vi "PythonNode_AddTwoDoubles_timed.vi"() -> ()   [LabVIEW 2020]
doc: "This example demonstrates how to call a Python function and pass doubles as arguments. It uses a python function to compute the sum of two doubles."
uses:
  Program Files (x86)/National Instruments/LabVIEW 2020/examples/Connectivity/Python/support/PythonVersionsEnum.ctl
  <vilib>/Utility/High Resolution Relative Seconds.vi
panel:
  out "Time (us)":dbl
  out "Time (ms)":dbl format="%_19f"
  out "error out":errorcluster
  out "a + b":dbl
  in  "b":dbl=1.0
  in  "a":dbl=41.0
  in  "error in (no error)":errorcluster
  in  "Python version":T1
  # "Overview: Demonstrates how to call a Python function and pass doubles as arguments.\nRequirements: Python 2.7 or 3.6 with the same bitness as LabVIEW.\nInstructions:\n1. Set the Python version to the version of Python you want to execute code in.\n2. Run the VI. You should see the result of adding \"a\" and \"b\" in the indicator \"a + b\".\n3. See comments on the block diagram of this VI and in \"ExamplePythonModule.py\" for more information about how the call python node passes arguments and handles return values."
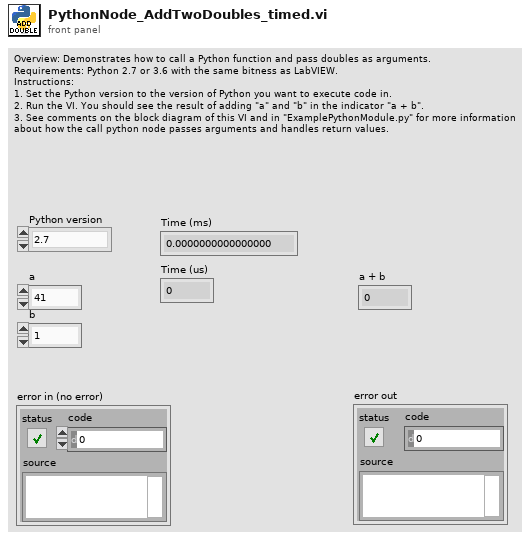
[diagram p1: front panel]
types:
  T1 = typedef "PythonVersionsEnum.ctl" = enum16{"2.7", "3.6"}
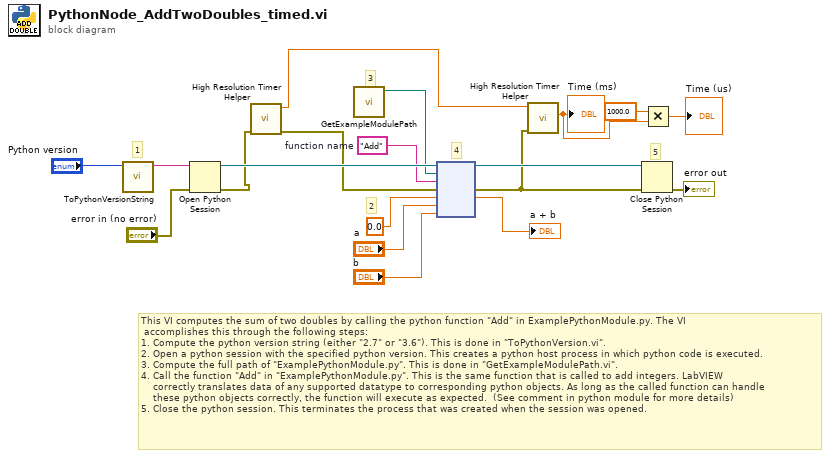
[diagram p0: block diagram]
diagram:
  w14 = "Add"  # function name
  # "5"
  # "4"
  # "2"
  # "3"
  # "1"
  # "This VI computes the sum of two doubles by calling the python function \"Add\" in ExamplePythonModule.py. The VI\n accomplishes this through the following steps:\n1. Compute the python version string (either \"2.7\" or \"3.6\"). This is done in \"ToPythonVersion.vi\". \n2. Open a python session with the specified python version. This creates a python host process in which python code is executed.\n3. Compute the full path of \"ExamplePythonModule.py\". This is done in \"GetExampleModulePath.vi\".\n4. Call the function \"Add\" in \"ExamplePythonModule.py\". This is the same function that is called to add integers. LabVIEW \n    correctly translates data of any supported datatype to corresponding python objects. As long as the called function can handle\n    these python objects correctly, the function will execute as expected.  (See comment in python module for more details)\n5. Close the python session. This terminates the process that was created when the session was opened."
  n1 = call "ToPythonVersionString.vi"("python version"="Python version") -> ("python version string"=w19:string)  [unwired: 10 in]
  n2 = Open Python Session(python version=w19, 3:"error in (no error)") -> (session out=w16:refnum<k35>, error out=w7:errorcluster)  [unwired: 1 in]
  n3 = call "High Resolution Timer Helper.vi"("error in (no error)"=w7) -> ("error out"=w1:errorcluster, "Current Time"=w5:dbl)  [unwired: 8 in, 1 out]
  n4 = call "GetExampleModulePath.vi"() -> ("module path"=w15:path)  [unwired: 11 in]
  n5 = node(w16, w15, w14, w1, 0.0 ("a"), "a", "b") -> (w13:refnum<k35>, w6:errorcluster, →"a + b":dbl)  [unwired: 2 in, 2 out]
  n6 = call "High Resolution Timer Helper.vi"("error in (no error)"=w6, "Previous Time"=w5) -> ("Time Difference (ms)"=w4:dbl)  [unwired: 7 in, 2 out]
  "Time (ms)" <- w4
  n7 = Close Python Session(session in=w13, error in=w6) -> (11:→"error out":errorcluster)
  n8 = Multiply(x=1000.0, y=w4) -> (x*y=→"Time (us)":dbl)
